vi "Play.vi"() -> ()   [LabVIEW 2020]
doc: "Use this template to build a producer/consumer design pattern with events to produce queue items. Use this design pattern instead of the User Interface Event Handler pattern for user interfaces when you want to execute code asynchronously in response to an event without slowing the user interface responsiveness."
uses:
  TypeDef/display.ctl
  TypeDef/tiles.ctl
  Support/MetronomeData.ctl
  TypeDef/game-data.ctl
  TypeDef/tiles-key.ctl
  Support/MessageQueue/QueueRef.ctl
  <vilib>/Utility/error.llb/Error Cluster From Error Code.vi
  <vilib>/ErrorRing/Error Ring.xnode
  Support/MessageQueue/MessageQueue.lvlib
panel:
  out "Display":T1
  in  "Right Button":bool
  in  "Left Button":bool
  in  "Down Button":bool
  in  "Up Button":bool
  in  "Start":bool
  in  "Exit":bool
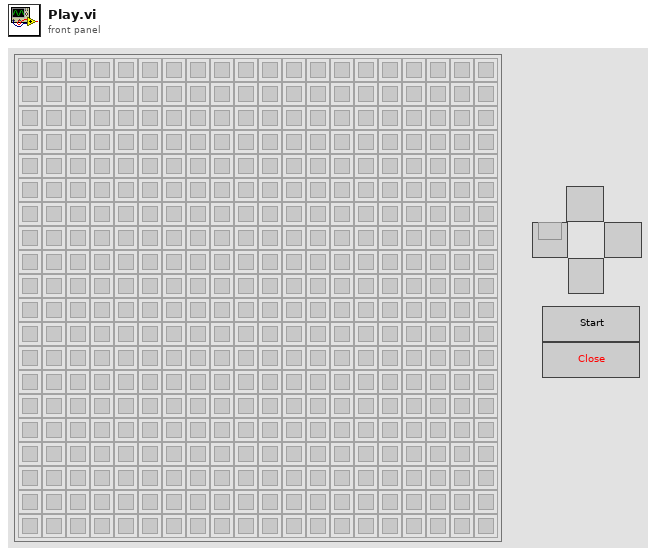
[diagram p1: front panel]
types:
  T1 = typedef "display.ctl" = T2[][]
  T2 = typedef "tiles.ctl" = u16
  T3 = typedef "game-data.ctl" = cluster{"Board":T4[][], "Target":cluster{"X":i32, "Y":i32, "Frame":i8}, "Head":cluster{"X":i32, "Y":i32}, "Tail":cluster{"X":i32, "Y":i32}}
  T4 = typedef "tiles-key.ctl" = enum16{"ground", "wall", "head (right)", "head (up)", "head (left)", "head (down)", "L-turn (right-up)", "L-turn (up-left)", "L-turn (left-down)", "L-turn (down-right)", "body (right)", "body (up)", "body (left)", "body (down)", "R-turn (right-down)", "R-turn (up-right)", "R-turn (left-up)", "R-turn (down-left)", "tail (right)", "tail (up)", "tail (left)", "tail (down)", "dead head (right)", "dead head (up)", "dead head (left)", "dead head (down)", "dead L-turn (right-up)", "dead L-turn (up-left)", "dead L-turn (left-down)", "dead L-turn (down-right)", "dead body (right)", "dead body (up)", "dead body (left)", "dead body (down)", "dead R-turn (right-down)", "dead R-turn (up-right)", "dead R-turn (left-up)", "dead R-turn (down-left)", "dead tail (right)", "dead tail (up)", "dead tail (left)", "dead tail (down)", "target red", "target blue", "target yellow", "target green"}
  T5 = typedef "MetronomeData.ctl" = cluster{"Interval":i32, "Message":string}
  T6 = typedef "MessageQueue.lvlib/QueueRef.ctl" = refnum<queue>
  T7 = cluster{"Data Handler":T6, "Blinker":T6, "Steps":T6, "Stop Event":refnum<user-event>}
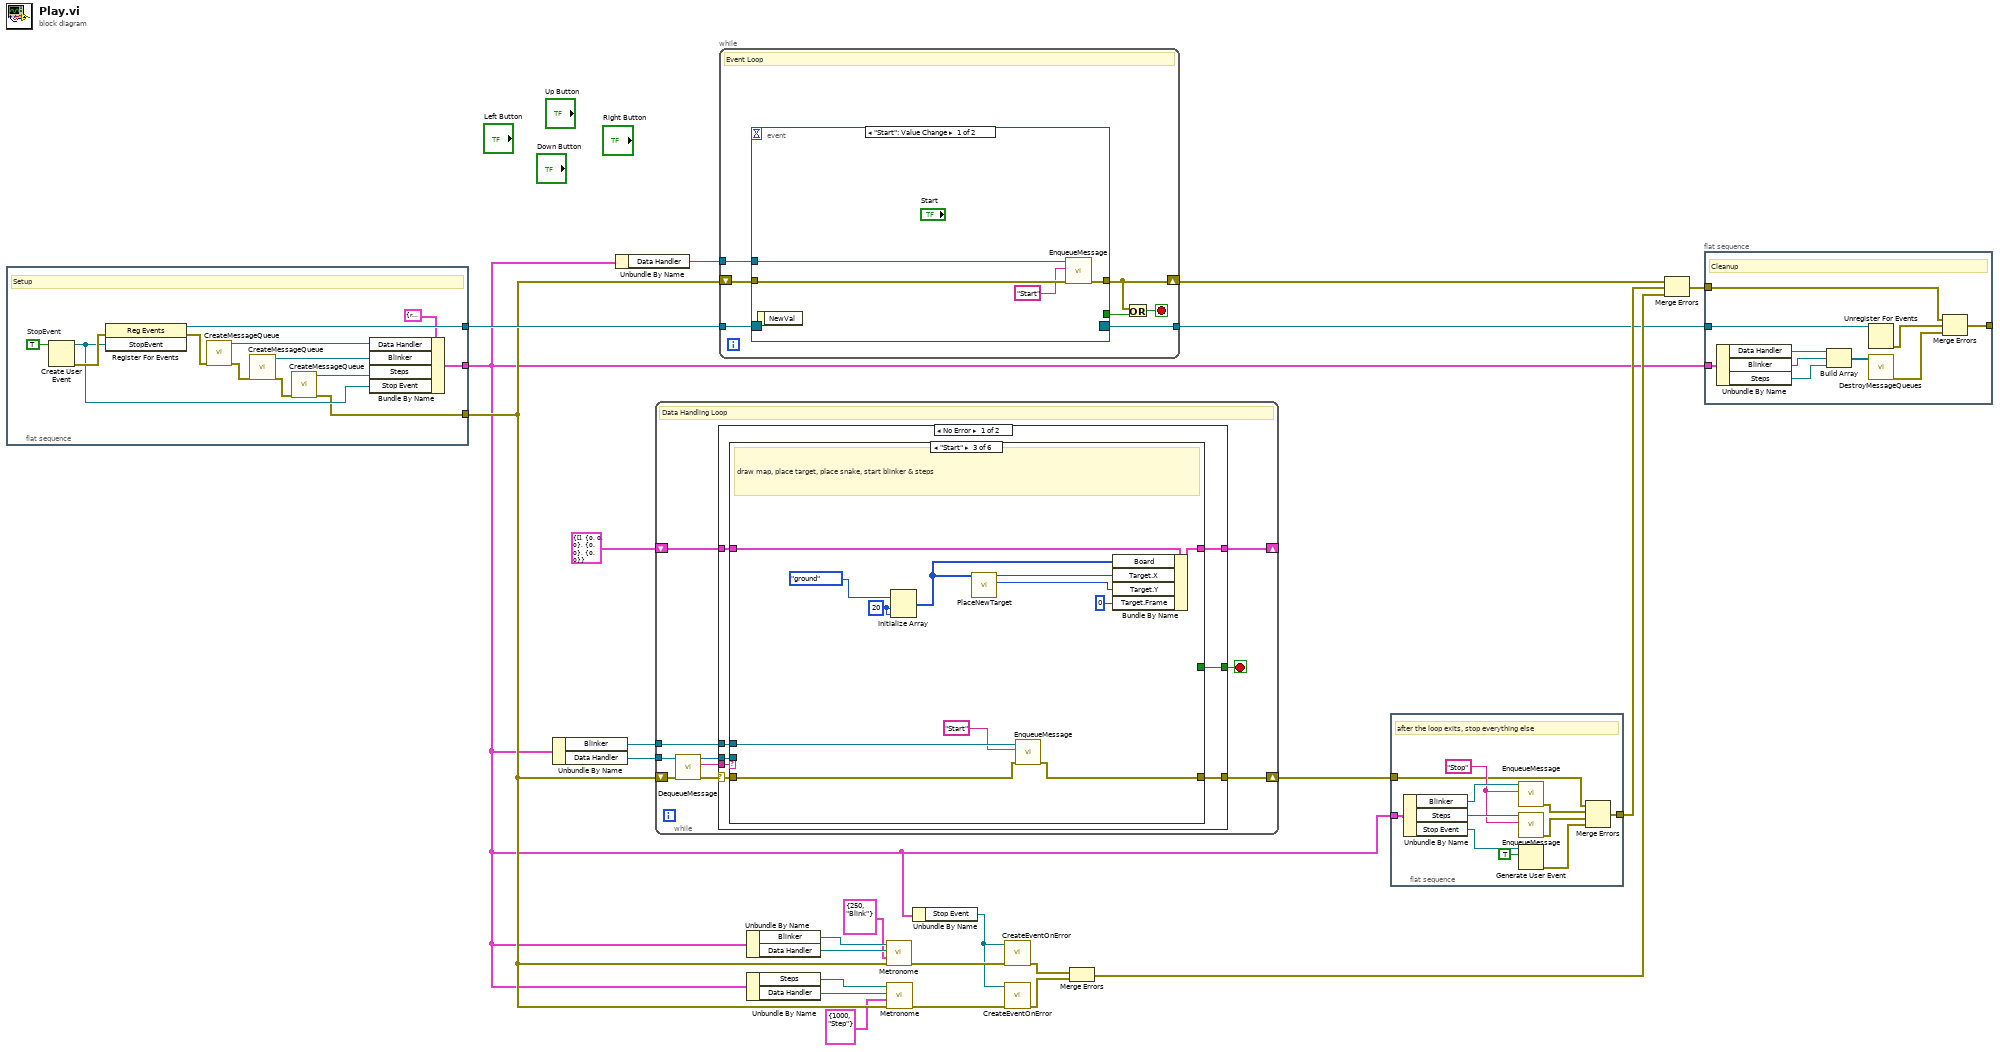
[diagram p0: block diagram]
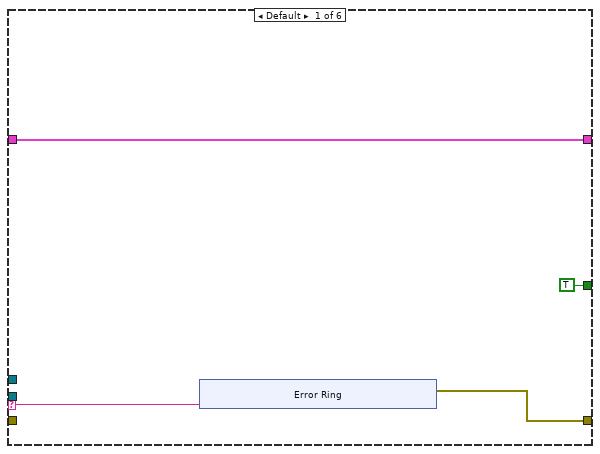
[diagram p2: hidden frame]
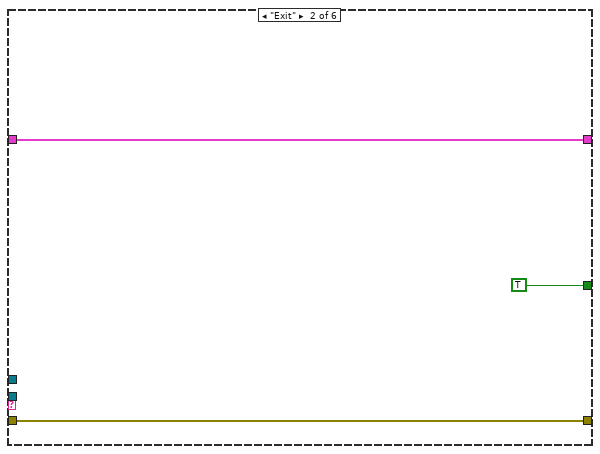
[diagram p3: hidden frame]
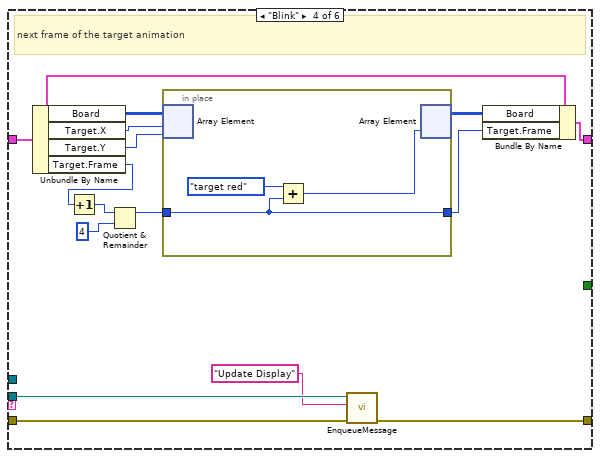
[diagram p4: hidden frame]
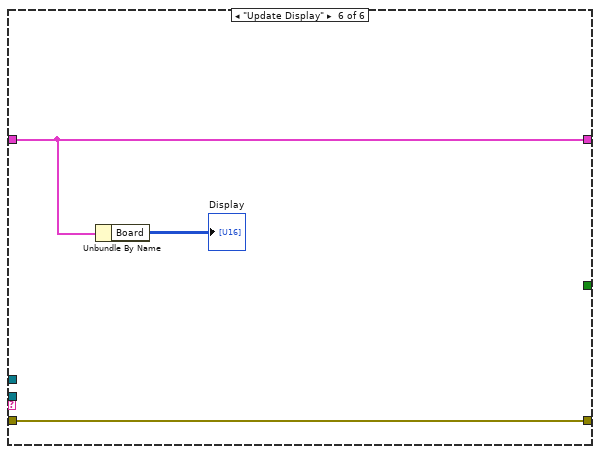
[diagram p6: hidden frame]
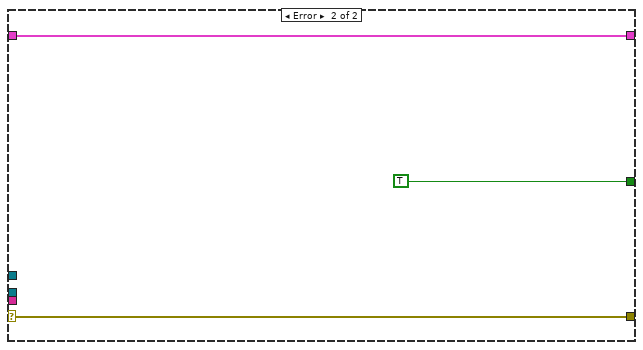
[diagram p7: hidden frame]
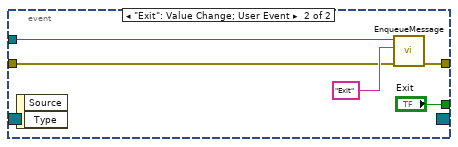
[diagram p8: hidden frame]
diagram:
  n1 = flat-sequence {
    tunnel: [w32] -> w24
    tunnel: [w26] -> w17
    tunnel: [w25] -> w5
    frame #0 {
      w28 = TRUE  # StopEvent
      # "Setup"
      n2 = Create User Event(user event datatype=w28) -> (user event=w29:refnum<user-event>, error out=w31:errorcluster)  [unwired: 1 in]
      n3 = register-events(error in=w31, w29) -> (reference out=w32:refnum<event-registration>, error out=w30:errorcluster)  [unwired: 1 in]
      n4 = call "CreateMessageQueue.vi"("error in (no error)"=w30) -> ("error out"=w34:errorcluster, "queue out"=w37:T6)  [unwired: 9 in]
      n5 = call "CreateMessageQueue.vi"("error in (no error)"=w34) -> ("error out"=w33:errorcluster, "queue out"=w36:T6)  [unwired: 9 in]
      n6 = call "CreateMessageQueue.vi"("error in (no error)"=w33) -> ("error out"=w26:errorcluster, "queue out"=w35:T6)  [unwired: 9 in]
      n7 = Bundle By Name(cluster=T7 {"Data Handler"=refnum, "Blinker"=refnum, "Steps"=refnum, "Stop Event"=refnum} ("output cluster"), "Data Handler"=w37, "Blinker"=w36, "Steps"=w35, "Stop Event"=w29) -> (w25:T7)
    }
  }
  n8 = Unbundle By Name(w5) -> ("Blinker"=w1:T6, "Data Handler"=w22:T6)
  n9 = Unbundle By Name(w5) -> ("Data Handler"=w23:T6)
  n10 = while {
    shift-right: [w43] -> w9
    shift-left: w17 -> [w44]
    tunnel: w22 -> [w42]
    shift-right: [w40] -> _
    shift-left: T3 {"Board"=[], "Target"={"X"=0, "Y"=0, "Frame"=0}, "Head"={"X"=0, "Y"=0}, "Tail"={"X"=0, "Y"=0}} ("Game Data") -> [w41]
    tunnel: w1 -> [w39]
    stop <- w45 stop-if-true
    # "Data Handling Loop"
    n11 = call "DequeueMessage.vi"("error in (no error)"=w44, "queue in"=w42) -> ("error out"=w47:errorcluster, "Message"=w46:string, "queue out (copy)"=w38:T6)  [unwired: 6 in, 1 out]
    n12 = case shown="No Error" w47 {
      selector: w47 -> [w52 w106]
      tunnel: w46 -> [w55 _]
      tunnel: [w54 TRUE] -> w45
      tunnel: [w53 w106] -> w43
      tunnel: w41 -> [w51 w105]
      tunnel: [w50 w105] -> w40
      tunnel: w39 -> [w49 _]
      tunnel: w38 -> [w48 _]
      frame No Error {
        n13 = case shown="\"Start\"" w55 {
          selector: w55 -> [w58 _ _ _ _ _]
          tunnel: [TRUE TRUE _ _ _ _] -> w54
          tunnel: [w57 w68 w74 w93 w101 w104] -> w53
          tunnel: w52 -> [_ w68 w75 w94 w101 w104]
          tunnel: w51 -> [w56 w67 w80 w96 w100 w103]
          tunnel: [w56 w67 w81 w95 w100 w103] -> w50
          tunnel: w49 -> [_ _ w76 _ _ _]
          tunnel: w48 -> [_ _ _ w92 _ _]
          frame Default {
            n14 = xnode "Error Ring"("parameter 0"=w58) -> ("error out"=w57:errorcluster)
          }
          frame "Exit" {
          }
          frame "Start" {
            w78 = 20 ("dimension size")
            # "draw map, place target, place snake, start blinker & steps"
            n15 = Initialize Array(tiles-key."ground" ("Tiles-key"), w78, w78) -> (w70:T4[][])
            n16 = call "PlaceNewTarget.vi"("Board"=w70) -> ("Position Y"=w71:i32, "Position X"=w72:i32)  [unwired: 8 in, 1 out]
            n17 = call "EnqueueMessage.vi"("error in (no error)"=w75, "Message"="Start", "queue in"=w76) -> ("error out"=w74:errorcluster)  [unwired: 7 in, 1 out]
            n18 = Bundle By Name(cluster=w80, "Board"=w70, "Target.X"=w72, "Target.Y"=w71, "Target.Frame"=i8 0) -> (w81:T3)
          }
          frame "Blink" {
            # "next frame of the target animation"
            n19 = Unbundle By Name(w96) -> ("Board"=w88:T4[][], "Target.X"=w87:i32, "Target.Y"=w84:i32, "Target.Frame"=w82:i8)
            n20 = Increment(x=w82) -> (x+1=w90:i8)
            n21 = Quotient & Remainder(x=w90, y=i8 4) -> (x-y*floor(x/y)=w86:i8)  [unwired: 1 out]
            n22 = in-place {
              in-place-border: w86 -> [w98]
              in-place-border: [w98] -> w83
              n23 = in-place-array #1(w88, w87, w84) -> ()  [unwired: 1 out]
              n24 = Add(x=tiles-key."target red" ("Tiles-key"), y=w98) -> (x+y=w97:u16)
              n25 = in-place-array #1(w97) -> (w85:T4[][])  [unwired: 2 out]
            }
            n26 = call "EnqueueMessage.vi"("error in (no error)"=w94, "Message"="Update Display", "queue in"=w92) -> ("error out"=w93:errorcluster)  [unwired: 7 in, 1 out]
            n27 = Bundle By Name(cluster=w96, "Board"=w85, "Target.Frame"=w83) -> (w95:T3)
          }
          frame "Step" {
            # "move snake one step forward\n(resolving direction, colision check, target acqired check)"
          }
          frame "Update Display" {
            n28 = Unbundle By Name(w103) -> ("Board"=→"Display":T4[][])
          }
        }
      }
      frame Error {
      }
    }
  }
  n29 = while {
    shift-right: [w111] -> w6
    shift-left: w17 -> [w114]
    tunnel: w24 -> [w110]
    tunnel: w23 -> [w109]
    tunnel: [w108] -> w4
    stop <- w112 stop-if-true
    # "Event Loop"
    n30 = event shown="[0] \"Start\": Value Change" {
      selector: w110 -> [_ _]
      dyn-events: [_ _] -> w108
      timeout: _ -> [_ _]
      tunnel: w114 -> [w118 w121]
      tunnel: [w117 w120] -> w111
      tunnel: [_ "Exit"] -> w113
      tunnel: w109 -> [w116 w119]
      event "Start": Value Change {
        n31 = event-data() -> ()  [unwired: 1 in, 1 out]
        n32 = call "EnqueueMessage.vi"("error in (no error)"=w118, "Message"="Start" ("element"), "queue in"=w116) -> ("error out"=w117:errorcluster)  [unwired: 7 in, 1 out]
      }
      event "Exit": Value Change; User Event {
        n33 = event-data() -> ()  [unwired: 1 in, 2 out]
        n34 = call "EnqueueMessage.vi"("error in (no error)"=w121, "Message"="Exit" ("element"), "queue in"=w119) -> ("error out"=w120:errorcluster)  [unwired: 7 in, 1 out]
      }
    }
    n35 = Or(x=w111, y=w113) -> (x .or. y?=w112:bool)
  }
  n36 = Unbundle By Name(w5) -> ("Blinker"=w21:T6, "Data Handler"=w20:T6)
  n37 = Unbundle By Name(w5) -> ("Steps"=w18:T6, "Data Handler"=w19:T6)
  n38 = call "Metronome.vi"("error in (no error)"=w17, "MetronomeData"=T5 {"Interval"=250, "Message"="Blink"}, "Queue in (write)"=w20, "Queue in (read)"=w21) -> ("error out"=w14:errorcluster)  [unwired: 5 in, 2 out]
  n39 = call "Metronome.vi"("error in (no error)"=w17, "MetronomeData"=T5 {"Interval"=1000, "Message"="Step"}, "Queue in (write)"=w19, "Queue in (read)"=w18) -> ("error out"=w13:errorcluster)  [unwired: 5 in, 2 out]
  n40 = Unbundle By Name(w5) -> ("Stop Event"=w12:refnum<user-event>)
  n41 = call "CreateEventOnError.vi"("error in (no error)"=w14, "User Event in"=w12) -> ("error out"=w11:errorcluster)  [unwired: 9 in]
  n42 = call "CreateEventOnError.vi"("error in (no error)"=w13, "User Event in"=w12) -> ("error out"=w10:errorcluster)  [unwired: 9 in]
  n43 = Merge Errors(w11, w10) -> (w7:errorcluster)
  n44 = flat-sequence {
    tunnel: w5 -> [w134]
    tunnel: w9 -> [w128]
    tunnel: [w124] -> w8
    frame #0 {
      w131 = "Stop" ("element")
      # "after the loop exits, stop everything else"
      n45 = Unbundle By Name(w134) -> ("Blinker"=w133:T6, "Steps"=w132:T6, "Stop Event"=w130:refnum<user-event>)
      n46 = call "EnqueueMessage.vi"("Message"=w131, "queue in"=w133) -> ("error out"=w127:errorcluster)  [unwired: 8 in, 1 out]
      n47 = call "EnqueueMessage.vi"("Message"=w131, "queue in"=w132) -> ("error out"=w126:errorcluster)  [unwired: 8 in, 1 out]
      n48 = Generate User Event(user event=w130, event data cluster=TRUE ("event data")) -> (error out=w125:errorcluster)  [unwired: 2 in, 1 out]
      n49 = Merge Errors(w128, w127, w126, w125) -> (w124:errorcluster)
    }
  }
  n50 = Merge Errors(w6, w8, w7) -> (w3:errorcluster)
  n51 = flat-sequence {
    tunnel: w5 -> [w144]
    tunnel: w4 -> [w139]
    tunnel: w3 -> [w138]
    tunnel: [w135] -> _
    frame #0 {
      # "Cleanup"
      n52 = Unbundle By Name(w144) -> ("Data Handler"=w143:T6, "Blinker"=w142:T6, "Steps"=w141:T6)
      n53 = Build Array(w143, w142, w141) -> (w140:T6[])
      n54 = Unregister For Events(event registration refnum=w139) -> (error out=w137:errorcluster)  [unwired: 1 in]
      n55 = call "DestroyMessageQueues.vi"("queue in"=w140) -> ("error out"=w136:errorcluster)  [unwired: 10 in]
      n56 = Merge Errors(w138, w137, w136) -> (w135:errorcluster)
    }
  }
